vi "Entrada Digital LED's.vi"() -> ()   [LabVIEW 2023]
uses:
  <vilib>/Instr/_visa.llb/VISA Configure Serial Port (Instr).vi
panel:
  out "LED 4":bool
  out "LED 3":bool
  out "LED 2":bool
  in  "stop":bool
  in  "ENTRADA COM":refnum<visa-resource-name>
  out "LED":bool
  # "ENTRADA DIGITAL"
  # "ENTRADAS DIGITALES"
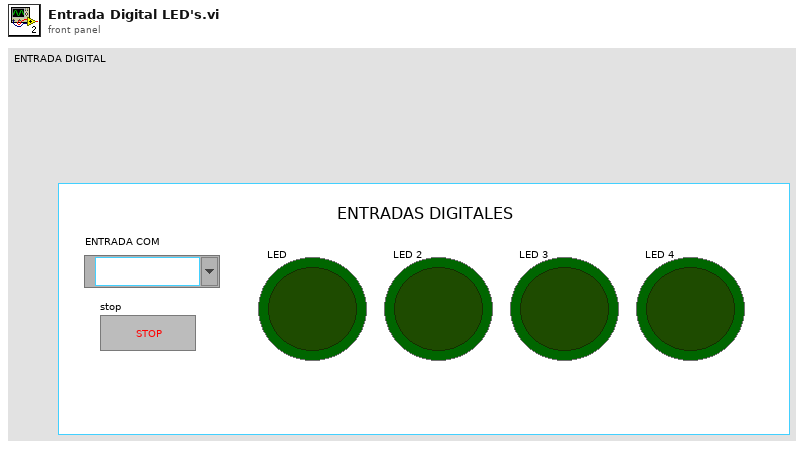
[diagram p1: front panel]
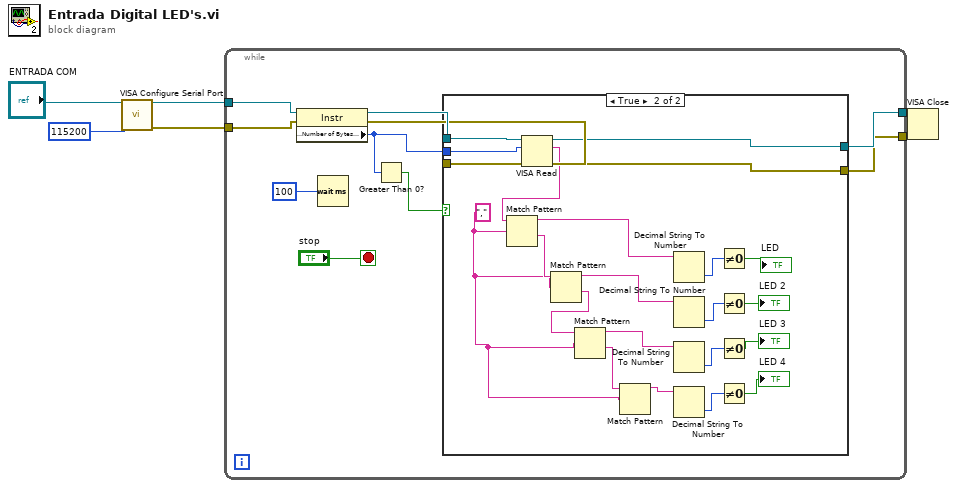
[diagram p0: block diagram]
diagram:
  n1 = call-poly "VISA Configure Serial Port"("VISA resource name"="ENTRADA COM", "baud rate (9600)"=u32 115200) -> ("VISA resource name out"=w2:refnum<visa-resource-name>, "error out"=w1:errorcluster)  [unwired: 12 in]
  n2 = while {
    tunnel: [w14] -> w4
    tunnel: [w13] -> w3
    tunnel: w2 -> [w10]
    tunnel: w1 -> [w9]
    stop <- "stop" stop-if-true
    n3 = property class="Instr"(reference=w10, error in=w9) -> (reference out=w12:refnum<visa-resource-name>, error out=w11:errorcluster, "Serial Settings:Number of Bytes at Serial Port"=w7:u32)
    n4 = Wait (ms)(milliseconds to wait=u32 100) -> ()  [unwired: 1 out]
    n5 = Greater Than 0?(x=w7) -> (x > 0?=w8:bool)
    n6 = case shown="True" w8 {
      tunnel: [w17 w40] -> w14
      tunnel: [w18 w39] -> w13
      tunnel: w12 -> [w17 w38]
      tunnel: w11 -> [w18 w37]
      tunnel: w7 -> [_ w36]
      frame False {
      }
      frame True {
        w21 = "," ("regular expression")
        n7 = VISA Read(VISA resource name=w38, byte count=w36, error in (no error)=w37) -> (VISA resource name out=w40:refnum<visa-resource-name>, read buffer=w19:string, error out=w39:errorcluster)  [unwired: 1 out]
        n8 = Match Pattern(string=w19, regular expression=w21) -> (before substring=w34:string, after substring=w32:string)  [unwired: 1 in, 2 out]
        n9 = Match Pattern(string=w32, regular expression=w21) -> (before substring=w29:string, after substring=w23:string)  [unwired: 1 in, 2 out]
        n10 = Match Pattern(string=w23, regular expression=w21) -> (before substring=w24:string, after substring=w22:string)  [unwired: 1 in, 2 out]
        n11 = Match Pattern(string=w22, regular expression=w21) -> (before substring=w20:string)  [unwired: 1 in, 3 out]
        n12 = Decimal String To Number(string=w34) -> (number=w33:i32)  [unwired: 2 in, 1 out]
        n13 = Decimal String To Number(string=w29) -> (number=w31:i32)  [unwired: 2 in, 1 out]
        n14 = Decimal String To Number(string=w24) -> (number=w28:i32)  [unwired: 2 in, 1 out]
        n15 = Decimal String To Number(string=w20) -> (number=w27:i32)  [unwired: 2 in, 1 out]
        n16 = Not Equal To 0?(x=w33) -> (x != 0?=→"LED":bool)
        n17 = Not Equal To 0?(x=w31) -> (x != 0?=→"LED 2":bool)
        n18 = Not Equal To 0?(x=w28) -> (x != 0?=→"LED 3":bool)
        n19 = Not Equal To 0?(x=w27) -> (x != 0?=→"LED 4":bool)
      }
    }
  }
  n20 = VISA Close(VISA resource name=w4, error in (no error)=w3) -> ()  [unwired: 1 out]
